vi "Periodic Tasks.vi"(8 "error in":errorcluster) -> ()   [LabVIEW 2019]
doc: "This VI runs in parallel to other tasks. It can contain as many user-defined periodic loops as you need. These can carry out PID or other sorts of timed response."
uses:
  <vilib>/Rock Robotics/WPI/Utilities/WPI_GetSetVariantRefNum.vi
  <vilib>/Rock Robotics/Network Tables/NT Write Number.vi
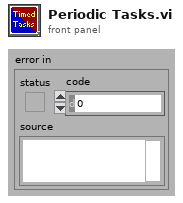
[diagram p1: front panel]
types:
  T1 = typedef "WPI_AnalogChannelDevRef.ctl" = cluster{"DevStatus":errorcluster, "Analog Channel":T2}
  T2 = typedef "FPGA_AIChannel.ctl" = enum8{"AI 0", "AI 1", "AI 2", "AI 3", "AI MXP 0", "AI MXP 1", "AI MXP 2", "AI MXP 3", "Invalid"}
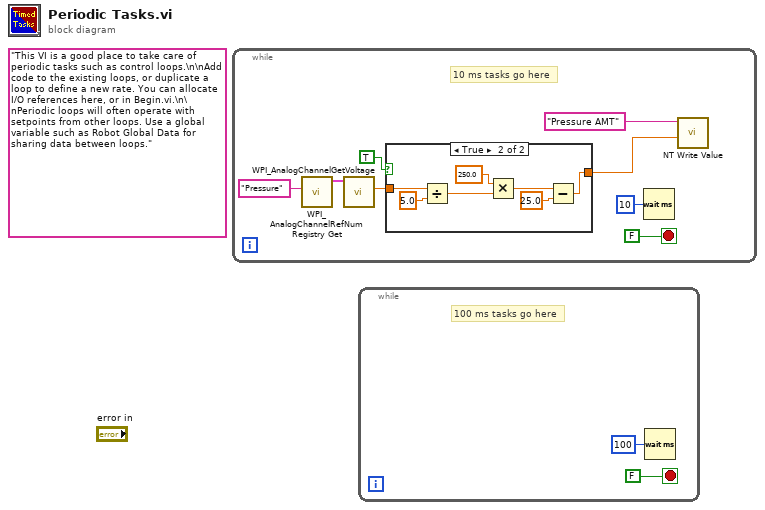
[diagram p0: block diagram]
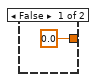
[diagram p2: hidden frame]
diagram:
  (unwired) "This VI is a good place to take care of periodic tasks such as control loops.\n\nAdd code to the existing loops, or duplicate a loop to define a new rate. You can allocate I/O references here, or in Begin.vi.\n\nPeriodic loops will often operate with setpoints from other loops. Use a global variable such as Robot Global Data for sharing data between loops."
  n1 = while {
    stop <- FALSE stop-if-true
    # "10 ms tasks go here"
    n2 = call <vilib>:"WPI_AnalogChannelRefNum Registry Get.vi"("refnum name"="Pressure") -> ("AIDeviceRef"=w4:T1)  [unwired: 9 in, 1 out]
    n3 = call <vilib>:"WPI_AnalogChannelGetVoltage.vi"("AIDeviceRef"=w4) -> ("Voltage"=w5:dbl)  [unwired: 8 in, 2 out]
    n4 = case shown="True" TRUE {
      tunnel: w5 -> [_ w11]
      tunnel: [0.0 w10] -> w6
      frame False {
      }
      frame True {
        n5 = Divide(x=w11, y=5.0) -> (x/y=w15:dbl)
        n6 = Multiply(x=250.0, y=w15) -> (x*y=w13:dbl)
        n7 = Subtract(x=w13, y=25.0) -> (x-y=w10:dbl)
      }
    }
    n8 = Wait (ms)(milliseconds to wait=u32 10) -> ()  [unwired: 1 out]
    n9 = call-poly <vilib>:"NT Write Value.vi"("Numeric"=w6, "Name"="Pressure AMT") -> ()  [unwired: 9 in, 1 out]
  }
  n10 = while {
    stop <- FALSE stop-if-true
    # "100 ms tasks go here"
    n11 = Wait (ms)(milliseconds to wait=u32 100) -> ()  [unwired: 1 out]
  }
